vi "Set Containers Notifications.vi"(7 "Ref Array":T1(array[cluster]), 8 "error in (no error)":errorcluster, 11 "Samples in":refnum<class "Samples.lvclass">) -> (0 "error out":errorcluster, 3 "Samples out":refnum<class "Samples.lvclass">)   [LabVIEW 2015, in "AMS UI.lvlib" / "Samples.lvclass"]
uses:
  Samples.lvclass
  Samples.lvclass/Samples.ctl
  <vilib>/lvdsc/NI_DSC.lvlib
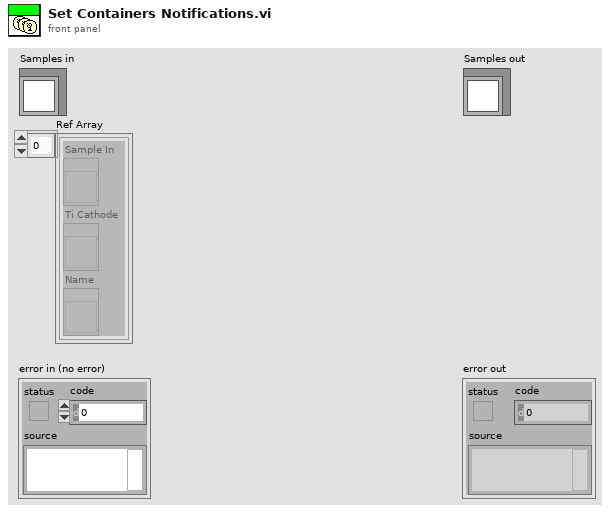
[diagram p1: front panel]
types:
  T1 = cluster{"Sample In":refnum<vi>, "Ti Cathode":refnum<vi>, "Name":refnum<vi>}[]
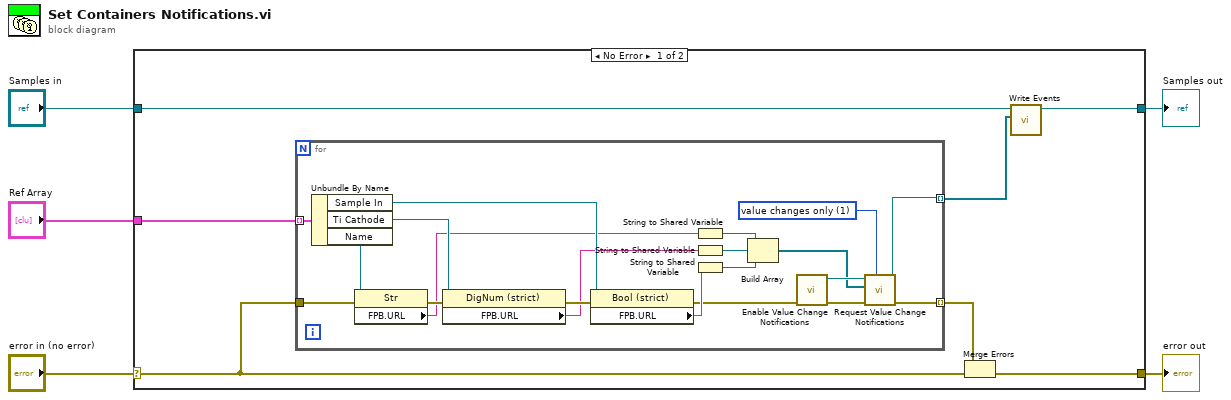
[diagram p0: block diagram]
diagram:
  n1 = case shown="No Error" "error in (no error)" {
    selector: "error in (no error)" -> [w11 w34]
    tunnel: [w8 w34] -> w4
    tunnel: [w10 w33] -> w2
    tunnel: "Samples in" -> [w7 w33]
    tunnel: "Ref Array" -> [w12 _]
    frame No Error {
      n2 = for {
        tunnel: w12 -> [w32] mode=indexing
        tunnel: w11 -> [w30]
        tunnel: [w13] -> w6 mode=indexing
        tunnel: [w17] -> w9 mode=indexing
        w16 = u16 1 items=["all changes", "value changes only"] ("request changes (all changes)")
        n3 = Unbundle By Name(w32) -> ("Sample In"=w26:refnum<vi>, "Ti Cathode"=w28:refnum<vi>, "Name"=w31:refnum<vi>)
        n4 = property class="Str"(reference=w31, error in=w30) -> (error out=w29:errorcluster, "FPB.URL"=w25:string)  [unwired: 1 out]
        n5 = property class="DigNum (strict)"(reference=w28, error in=w29) -> (error out=w27:errorcluster, "FPB.URL"=w24:string)  [unwired: 1 out]
        n6 = property class="Bool (strict)"(reference=w26, error in=w27) -> (error out=w21:errorcluster, "FPB.URL"=w23:string)  [unwired: 1 out]
        n7 = String to Shared Variable(0:w25) -> (2:w15:refnum<k21>)  [unwired: 1 out]
        n8 = String to Shared Variable(0:w24) -> (2:w14:refnum<k21>)  [unwired: 1 out]
        n9 = String to Shared Variable(0:w23) -> (2:w22:refnum<k21>)  [unwired: 1 out]
        n10 = Build Array(w15, w14, w22) -> (w18:refnum<k21>[])
        n11 = call <vilib>:"Enable Value Change Notifications.vi"("error in (no error)"=w21) -> ("error out"=w20:errorcluster, "shared variable value change notification"=w19:refnum<user-event>)  [unwired: 9 in]
        n12 = call <vilib>:"Request Value Change Notifications.vi"("request changes (all changes)"=w16, "error in (no error)"=w20, "shared variables"=w18, "notification refnum"=w19) -> ("error out"=w17:errorcluster, "shared variable value change notification"=w13:refnum<user-event>)  [unwired: 5 in, 1 out]
      }
      n13 = Merge Errors(w9, w11) -> (w8:errorcluster)
      n14 = call "Write Events.vi"("Events"=w6, "Samples in"=w7) -> ("Samples out"=w10:refnum<class "Samples.lvclass">)  [unwired: 9 in]
    }
    frame Error {
    }
  }
  "error out" <- w4
  "Samples out" <- w2
